vi "Plot Hyperbola.vi"(0 "Center Coordinates":cluster{"x":dbl, "y":dbl}, 2 "Rotation Angle (rad)":dbl format="%#_13g", 3 "Semimajor Axis (a)":dbl format="%#_13g", 5 "Distance to Focus (c)":dbl format="%#_13g") -> ()   [LabVIEW 2013]
uses:
  <vilib>/Analysis/baseanly.llb/A x Vector.vi
  <vilib>/gmath/NI_Gmath.lvlib
  <vilib>/Analysis/NI_AALBase.lvlib
panel:
  out "XY Graph":cluster{"X":dbl, "Y":dbl}[](graph)
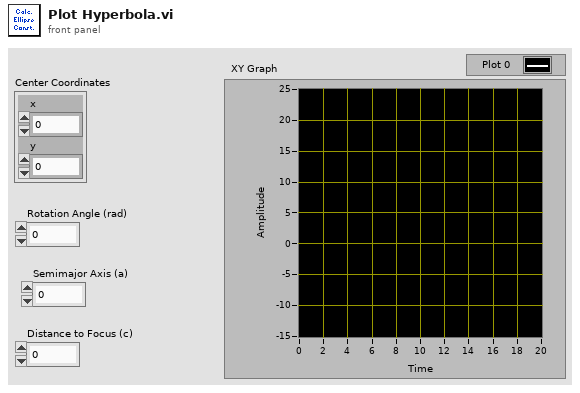
[diagram p1: front panel]
types:
  T1 = cluster{"A x Vector[0]":dbl, "A x Vector[1]":dbl}
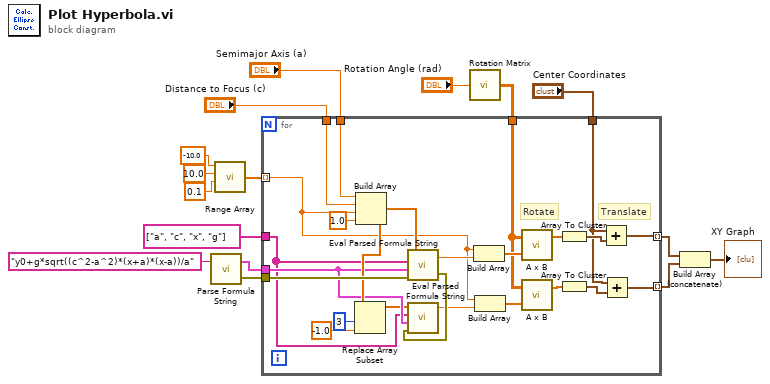
[diagram p0: block diagram]
diagram:
  n1 = call <vilib>:"Parse Formula String.vi"("formula"="y0+g*sqrt((c^2-a^2)*(x+a)*(x-a))/a") -> ("error out"=w16:errorcluster, "Parsed Formula"=w14:cluster{"Table":i32[][], "Y Values":dbl[]})  [unwired: 1 in]
  n2 = call "Range Array.vi"("Step"=0.1, "Stop"=10.0, "Start"=-10.0) -> ("Range"=w10:dbl[])  [unwired: 3 in]
  n3 = call "Rotation Matrix.vi"("Rotation Angle (rad)"="Rotation Angle (rad)") -> ("Rotation Matrix"=w2:dbl[][])  [unwired: 4 in]
  n4 = for {
    tunnel: w16 -> [w40]
    tunnel: w14 -> [w32]
    tunnel: w10 -> [w24] mode=indexing
    tunnel: string[] ["a", "c", "x", "g"] ("Variables") -> [w31]
    tunnel: "Semimajor Axis (a)" -> [w39]
    tunnel: "Distance to Focus (c)" -> [w38]
    tunnel: w2 -> [w25]
    tunnel: [w18] -> w6 mode=indexing
    tunnel: [w19] -> w5 mode=indexing
    tunnel: "Center Coordinates" -> [w17]
    # "Translate"
    # "Rotate"
    n5 = Build Array(w39, w38, w24, 1.0 ("element")) -> (w36:dbl[])
    n6 = Replace Array Subset(array=w36, new element=-1.0 ("new element/subarray"), index=3) -> (w30:dbl[])
    n7 = call <vilib>:"Eval Parsed Formula String.vi"("error in (no error)"=w40, "Parsed Formula"=w32, "Variables"=w31, "X Values"=w36) -> ("error out"=w33:errorcluster, "y value"=w29:dbl)
    n8 = call <vilib>:"Eval Parsed Formula String.vi"("error in (no error)"=w33, "Parsed Formula"=w32, "Variables"=w31, "X Values"=w30) -> ("y value"=w28:dbl)  [unwired: 1 out]
    n9 = Build Array(w24, w29) -> (w27:dbl[])
    n10 = Build Array(w24, w28) -> (w26:dbl[])
    n11 = call-poly <vilib>:"A x B.vi"("Vector"=w27, "A"=w25) -> ("A x Vector"=w23:dbl[])  [unwired: 1 out]
    n12 = call-poly <vilib>:"A x B.vi"("Vector"=w26, "A"=w25) -> ("A x Vector"=w22:dbl[])  [unwired: 1 out]
    n13 = Array To Cluster(array=w23) -> (cluster=w21:T1)
    n14 = Array To Cluster(array=w22) -> (cluster=w20:T1)
    n15 = Add(x=w17, y=w21) -> (x+y=w18:cluster{dbl, dbl})
    n16 = Add(x=w17, y=w20) -> (x+y=w19:cluster{dbl, dbl})
  }
  n17 = Build Array (concatenate)(w6, w5) -> (→"XY Graph":cluster{dbl, dbl}[])
